vi "AIT 664 Rx Message Ports Page.vi"(8 "error in (no error)":errorcluster, 11 "Node Ptr":T2 format="%.0x") -> (0 "error out":errorcluster)   [LabVIEW 2013, in "AIT 664 Custom Device.lvlib"]
uses:
  AIT 664 Custom Device.lvlib
  <vilib>/NI Veristand/Custom Device API/Custom Device Item Ref.ctl
  Controls/664 - Sampling Type.ctl
  Controls and Global/Global.vi
  <vilib>/NI Veristand/Custom Device API/Get Item Property (U32).vi
  <vilib>/NI Veristand/Custom Device API/Get Item Property (String).vi
  <vilib>/NI Veristand/Custom Device API/Get Item Property (Variant).vi
  <vilib>/NI Veristand/Custom Device API/Set Item Property (U32).vi
  <vilib>/NI Veristand/Custom Device API/Custom Device API.lvlib
panel:
  out "Buffer Depth":u32
  in  "Rx Rate (ms)":u32
  out "Destination UDP Port":u32
  out "Destination IP Address":string
  out "Source UDP Port":u32
  out "Source IP Address":string
  out "Sampling Type":T1
  out "Port Id":u32
  in  "Header":cluster{"Section Name":string}={"Section Name"="AIT 664 Rx Message Ports Page"}
  in  "Description":string
  out "Name":string
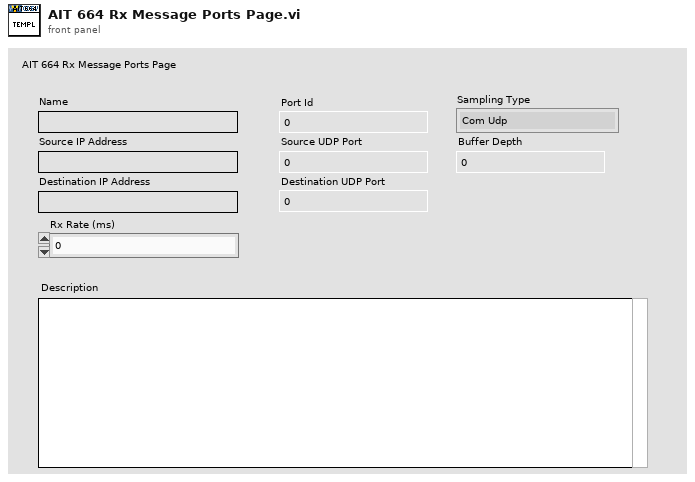
[diagram p1: front panel]
types:
  T1 = typedef "AIT 664 Custom Device.lvlib/664 - Sampling Type.ctl" = enum16{"Com Udp", "Com Udp Queuing", "Sap Udp", "Sap Ip", "Sap Mac", "Unknown"}
  T2 = typedef "Custom Device API.lvlib/Custom Device Item Ref.ctl" = u64
  T3 = typedef "Custom Device API.lvlib/Custom Device Item Info.ctl" = cluster{"Name":string, "Is Channel":bool, "GUID":string, "Is Waveform":bool}
  T4 = typedef "Custom Device API.lvlib/Custom Device Commands.ctl" = enum16{"Default", "Item renamed", "Shutdown", "Dynamic button pressed"}
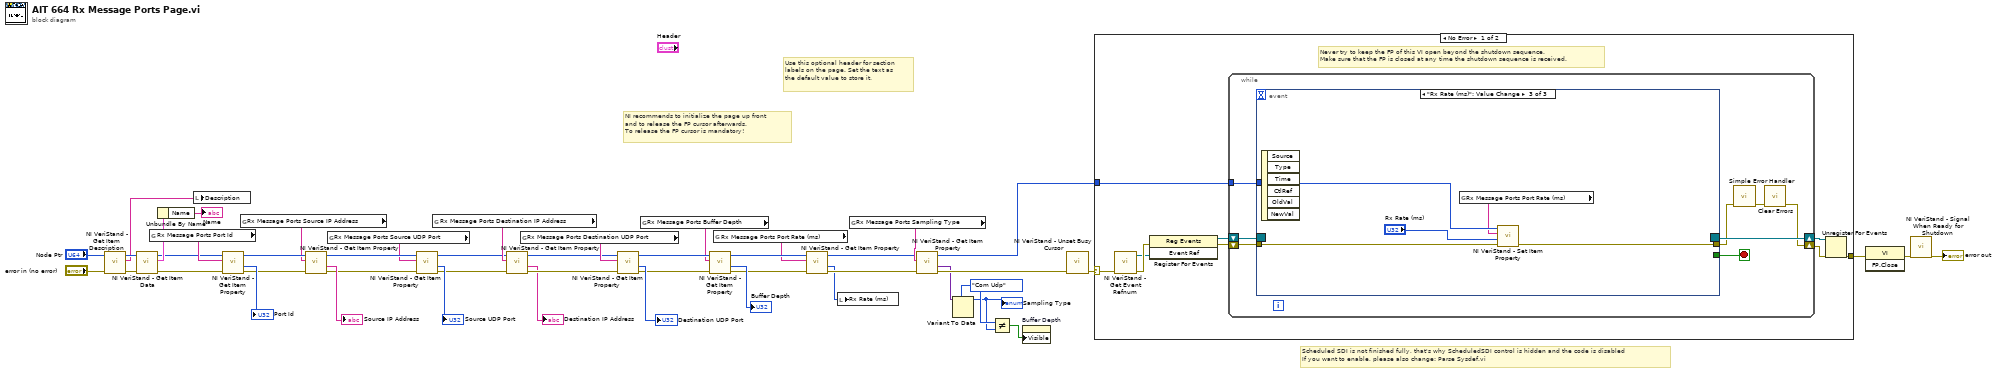
[diagram p0: block diagram]
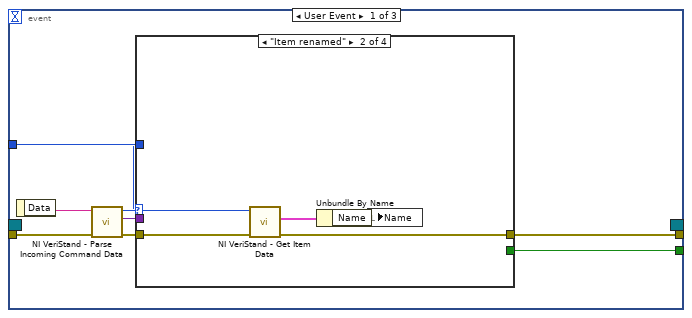
[diagram p2: hidden frame]
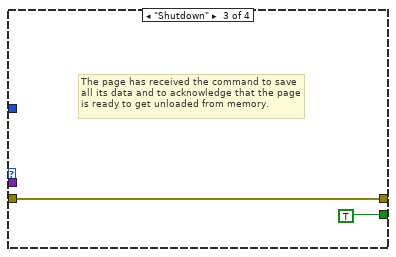
[diagram p4: hidden frame]
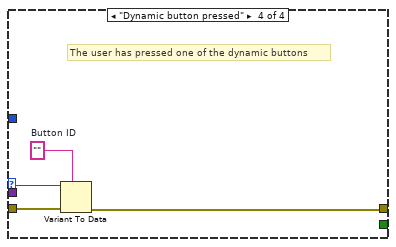
[diagram p5: hidden frame]
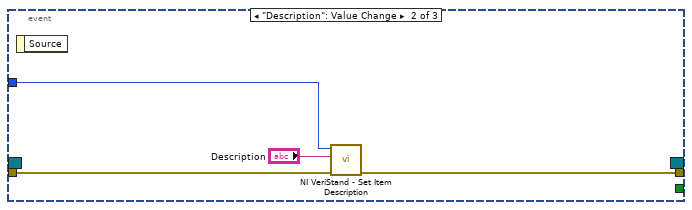
[diagram p6: hidden frame]
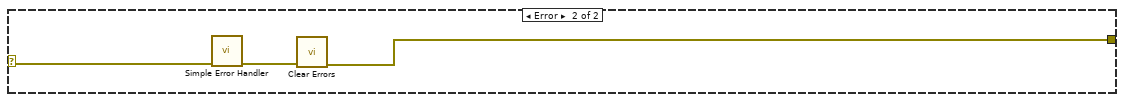
[diagram p7: hidden frame]
diagram:
  w3 = 664_-_Sampling_Type."Com Udp" ("Sampling Type")
  # "Scheduled SDI is not finished fully, that's why ScheduledSDI control is hidden and the code is disabled\nIf you want to enable, please also change: Parse Sysdef.vi"
  # "Use this optional header for section labels on the page. Set the text as the default value to store it."
  # "NI recommends to initialize the page up front\nand to release the FP cursor afterwards.\nTo release the FP cursor is mandatory!"
  n1 = call <vilib>:"NI VeriStand - Get Item Description.vi"("error in (no error)"="error in (no error)", "Item Ref in"="Node Ptr") -> ("error out"=w42:errorcluster, "Description"=w43:string, "Item Ref out"=w44:T2)  [unwired: 7 out]
  n2 = call <vilib>:"NI VeriStand - Get Item Data.vi"("error in (no error)"=w42, "Item Ref in"=w44) -> ("error out"=w35:errorcluster, "Item Info"=w41:T3, "Item Ref out"=w34:T2)  [unwired: 7 out]
  n3 = global read "Global.vi" "Rx Message Ports Port Id"() -> (w36:string)
  n4 = Unbundle By Name(w41) -> ("Name"=→"Name":string)
  n5 = local write "Description"(w43) -> ()
  n6 = call-poly <vilib>:"NI VeriStand - Get Item Property.vi"("error in (no error)"=w35, "Property Name"=w36, "Item Ref in"=w34) -> ("error out"=w29:errorcluster, "Value"=→"Port Id":u32, "Item Ref out"=w28:T2)  [unwired: 5 in, 1 out]
  n7 = global read "Global.vi" "Rx Message Ports Source IP Address"() -> (w27:string)
  n8 = call-poly <vilib>:"NI VeriStand - Get Item Property.vi"("error in (no error)"=w29, "Property Name"=w27, "Item Ref in"=w28) -> ("error out"=w25:errorcluster, "Value"=→"Source IP Address":string, "Item Ref out"=w24:T2)  [unwired: 5 in, 1 out]
  n9 = global read "Global.vi" "Rx Message Ports Source UDP Port"() -> (w22:string)
  n10 = call-poly <vilib>:"NI VeriStand - Get Item Property.vi"("error in (no error)"=w25, "Property Name"=w22, "Item Ref in"=w24) -> ("error out"=w17:errorcluster, "Value"=→"Source UDP Port":u32, "Item Ref out"=w16:T2)  [unwired: 5 in, 1 out]
  n11 = global read "Global.vi" "Rx Message Ports Destination IP Address"() -> (w18:string)
  n12 = call-poly <vilib>:"NI VeriStand - Get Item Property.vi"("error in (no error)"=w17, "Property Name"=w18, "Item Ref in"=w16) -> ("error out"=w19:errorcluster, "Value"=→"Destination IP Address":string, "Item Ref out"=w20:T2)  [unwired: 5 in, 1 out]
  n13 = global read "Global.vi" "Rx Message Ports Destination UDP Port"() -> (w21:string)
  n14 = call-poly <vilib>:"NI VeriStand - Get Item Property.vi"("error in (no error)"=w19, "Property Name"=w21, "Item Ref in"=w20) -> ("error out"=w13:errorcluster, "Value"=→"Destination UDP Port":u32, "Item Ref out"=w12:T2)  [unwired: 5 in, 1 out]
  n15 = global read "Global.vi" "Rx Message Ports Buffer Depth"() -> (w10:string)
  n16 = call-poly <vilib>:"NI VeriStand - Get Item Property.vi"("error in (no error)"=w13, "Property Name"=w10, "Item Ref in"=w12) -> ("error out"=w9:errorcluster, "Value"=→"Buffer Depth":u32, "Item Ref out"=w7:T2)  [unwired: 5 in, 1 out]
  n17 = global read "Global.vi" "Rx Message Ports Port Rate (ms)"() -> (w5:string)
  n18 = call-poly <vilib>:"NI VeriStand - Get Item Property.vi"("error in (no error)"=w9, "Property Name"=w5, "Item Ref in"=w7) -> ("error out"=w8:errorcluster, "Value"=w4:u32, "Item Ref out"=w6:T2)  [unwired: 5 in, 1 out]
  n19 = local write "Rx Rate (ms)"(w4) -> ()
  n20 = global read "Global.vi" "Rx Message Ports Sampling Type"() -> (w31:string)
  n21 = call-poly <vilib>:"NI VeriStand - Get Item Property.vi"("error in (no error)"=w8, "Property Name"=w31, "Item Ref in"=w6) -> ("error out"=w33:errorcluster, "Value"=w30:variant, "Item Ref out"=w32:T2)  [unwired: 5 in, 1 out]
  n22 = Variant To Data(type=w3, Variant=w30) -> (data=w2:T1)  [unwired: 1 in, 1 out]
  "Sampling Type" <- w2
  n23 = Not Equal?(x=w3, y=w2) -> (x != y?=w1:bool)
  n24 = property on="Buffer Depth" class="DigNum (strict)"("Visible"=w1) -> ()  [unwired: 2 in, 2 out]
  n25 = call <vilib>:"NI VeriStand - Unset Busy Cursor.vi"("error in (no error)"=w33) -> ("error out"=w45:errorcluster)  [unwired: 10 out]
  n26 = case shown="No Error" w45 {
    selector: w45 -> [w49 w97]
    tunnel: [w54 w95] -> w48
    tunnel: w32 -> [w50 _]
    frame No Error {
      # "Never try to keep the FP of this VI open beyond the shutdown sequence.\nMake sure that the FP is closed at any time the shutdown sequence is received."
      n27 = call <vilib>:"NI VeriStand - Get Event Refnum.vi"("error in (no error)"=w49) -> ("error out"=w57:errorcluster, "Event Ref"=w53:refnum<user-event>)  [unwired: 9 out]
      n28 = register-events(error in=w57, w53) -> (reference out=w51:refnum<event-registration>, error out=w52:errorcluster)  [unwired: 1 in]
      n29 = while {
        tunnel: w50 -> [w61]
        shift-right: [w58] -> w55
        shift-left: w52 -> [w64]
        shift-right: [w65] -> w56
        shift-left: w51 -> [w63]
        stop <- w62 stop-if-true
        n30 = event shown="[2] \"Rx Rate (ms)\": Value Change" {
          selector: w63 -> [_ _ _]
          dyn-events: [_ _ _] -> w65
          timeout: _ -> [_ _ _]
          tunnel: w64 -> [w73 w88 w93]
          tunnel: [w69 _ _] -> w62
          tunnel: [w68 w87 w92] -> w60
          tunnel: w61 -> [w67 w89 w94]
          event User Event {
            n31 = event-data() -> ("Data"=w72:string)  [unwired: 1 out]
            n32 = call <vilib>:"NI VeriStand - Parse Incoming Command Data.vi"("error in (no error)"=w73, "Incoming data"=w72) -> ("error out"=w71:errorcluster, "Outgoing data"=w66:variant, "Action"=w70:T4)  [unwired: 7 out]
            n33 = case shown="\"Item renamed\"" w70 {
              tunnel: w71 -> [w74 w79 w80 w85]
              tunnel: [_ _ TRUE _] -> w69
              tunnel: [w74 w76 w80 w82] -> w68
              tunnel: w67 -> [_ w78 _ _]
              tunnel: w66 -> [_ _ _ w84]
              frame "Default", Default {
              }
              frame "Item renamed" {
                n34 = call <vilib>:"NI VeriStand - Get Item Data.vi"("error in (no error)"=w79, "Item Ref in"=w78) -> ("error out"=w76:errorcluster, "Item Info"=w77:T3)  [unwired: 8 out]
                n35 = Unbundle By Name(w77) -> ("Name"=w75:string)
                n36 = local write "Name"(w75) -> ()
              }
              frame "Shutdown" {
                # "The page has received the command to save all its data and to acknowledge that the page is ready to get unloaded from memory."
              }
              frame "Dynamic button pressed" {
                w83 = ""  # Button ID
                # "The user has pressed one of the dynamic buttons"
                n37 = Variant To Data(error in=w85, type=w83, Variant=w84) -> (error out=w82:errorcluster)  [unwired: 1 out]
              }
            }
          }
          event "Description": Value Change {
            n38 = event-data() -> ()  [unwired: 2 out]
            n39 = call <vilib>:"NI VeriStand - Set Item Description.vi"("error in (no error)"=w88, "Description"="Description", "Item Ref in"=w89) -> ("error out"=w87:errorcluster)  [unwired: 8 out]
          }
          event "Rx Rate (ms)": Value Change {
            n40 = event-data() -> ()  [unwired: 7 out]
            n41 = global read "Global.vi" "Rx Message Ports Port Rate (ms)"() -> (w91:string)
            n42 = call-poly <vilib>:"NI VeriStand - Set Item Property.vi"("error in (no error)"=w93, "Value"="Rx Rate (ms)", "Property Name"=w91, "Item Ref in"=w94) -> ("error out"=w92:errorcluster)  [unwired: 5 in, 2 out]
          }
        }
        n43 = call <vilib>:"Simple Error Handler.vi"("error in (no error)"=w60) -> ("error out"=w59:errorcluster)  [unwired: 1 in, 7 out]
        n44 = call <vilib>:"Clear Errors.vi"("error in (no error)"=w59) -> ("error out"=w58:errorcluster)  [unwired: 6 out]
      }
      n45 = Unregister For Events(event registration refnum=w56, error in=w55) -> (error out=w54:errorcluster)
    }
    frame Error {
      n46 = call <vilib>:"Simple Error Handler.vi"("error in (no error)"=w97) -> ("error out"=w96:errorcluster)  [unwired: 1 in, 7 out]
      n47 = call <vilib>:"Clear Errors.vi"("error in (no error)"=w96) -> ("error out"=w95:errorcluster)  [unwired: 6 out]
    }
  }
  n48 = invoke class="VI" method="FP.Close"(error in=w48) -> (error out=w47:errorcluster)  [unwired: 2 in, 2 out]
  n49 = call <vilib>:"NI VeriStand - Signal When Ready for Shutdown.vi"("error in (no error)"=w47) -> ("error out"=→"error out":errorcluster)  [unwired: 10 out]
